vi "Get analysis parameters.vi"(6 "wait for reply (T)":bool=TRUE, 8 "error in":errorcluster) -> (0 "error out":errorcluster, 1 "timed out?":bool, 2 "Decimation":T2={"App"={"Dec"=1, "apply"=FALSE}, "Con"={"Dec"=1, "apply"=FALSE}, "Ret"={"Dec"=1, "apply"=FALSE}}, 3 "Contact":T3, 4 "Tau Delay (ms)":dbl, 5 "Savitzksky-Golay":T1)   [LabVIEW 2019, in "Main UI.lvlib"]
doc: "Gets the analysis parameters\n_____\nCreated using DQMH Event Scripter 6.1.0.128."
uses:
  Main UI.lvlib
  Main UI Shared/Decimation input --cluster.ctl
  Get analysis parameters Argument--cluster.ctl
  Get analysis parameters (Reply Payload)--cluster.ctl
  Main UI Shared/MAIN UI Shared.lvlib
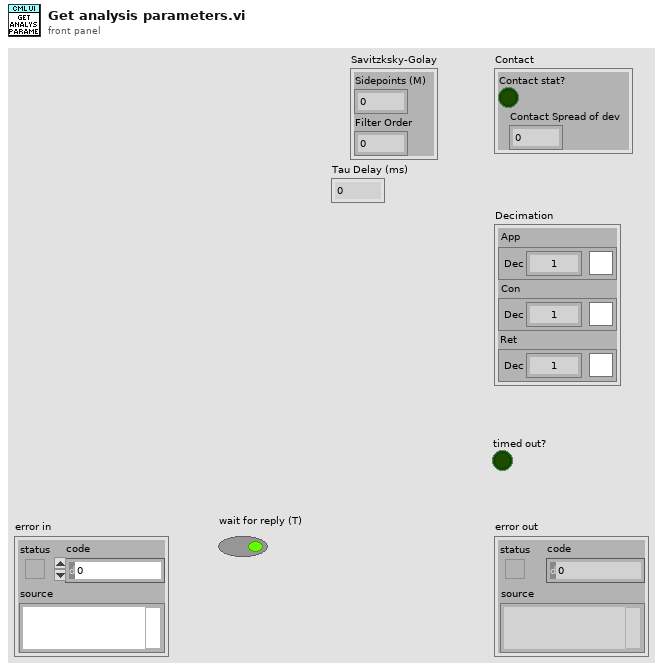
[diagram p1: front panel]
types:
  T1 = cluster{"Sidepoints (M)":dbl, "Filter Order":i32}
  T2 = typedef "MAIN UI Shared.lvlib/Decimation input --cluster.ctl" = cluster{"App":cluster{"Dec":i32, "apply":bool}, "Con":cluster{"Dec":i32, "apply":bool}, "Ret":cluster{"Dec":i32, "apply":bool}}
  T3 = cluster{"Contact stat?":bool, "Contact Spread of dev":dbl}
  T4 = typedef "Main UI.lvlib/Get analysis parameters Argument--cluster.ctl" = cluster{"Wait Notifier":refnum<notifier>, "wait for reply":bool}
  T5 = typedef "Main UI.lvlib/Request Events--cluster.ctl" = cluster{"Stop Module":refnum<user-event>, "Show Panel":refnum<user-event>, "Hide Panel":refnum<user-event>, "Get Module Execution Status":refnum<user-event>, "Show Diagram":refnum<user-event>, "Get analysis parameters":refnum<user-event>}
  T6 = typedef "Main UI.lvlib/Get analysis parameters (Reply Payload)--cluster.ctl" = cluster{"Contact":cluster{"Contact stat?":bool, "Contact Spread of dev":dbl}, "Decimation":T2, "Savitzksky-Golay":cluster{"Sidepoints (M)":dbl, "Filter Order":i32}, "Tau Delay (ms)":dbl, "error":errorcluster}
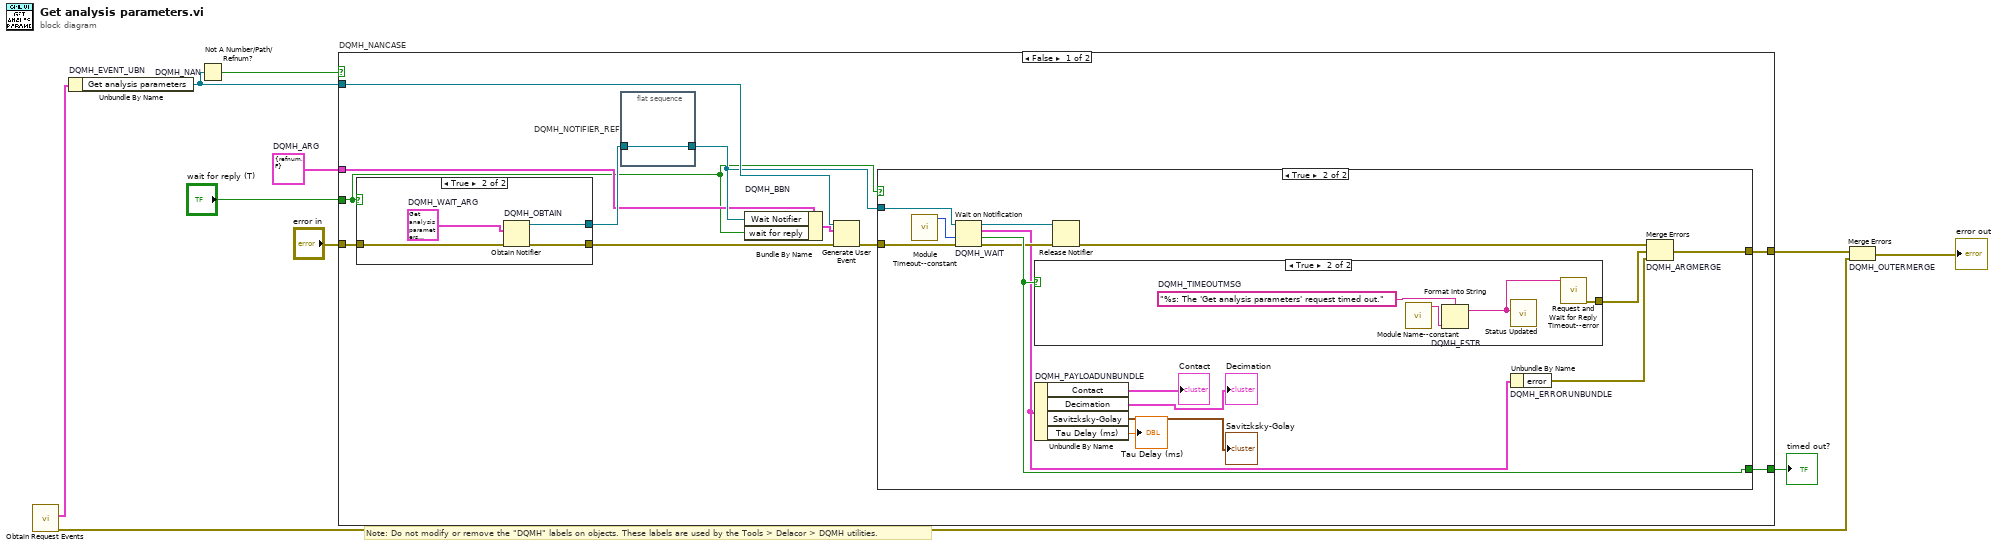
[diagram p0: block diagram]
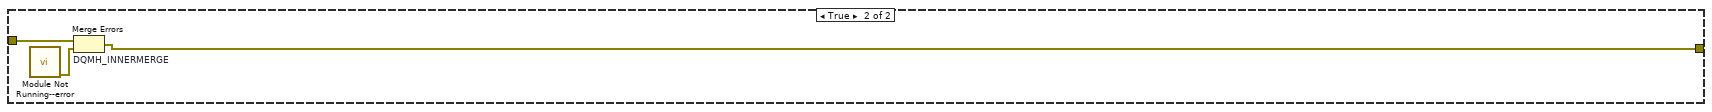
[diagram p5: hidden frame]
diagram:
  w4 = T4 {"Wait Notifier"=refnum, "wait for reply"=FALSE}  # DQMH_ARG
  # "Note: Do not modify or remove the \"DQMH\" labels on objects. These labels are used by the Tools > Delacor > DQMH utilities."
  n1 = call "Obtain Request Events.vi"() -> ("error out"=w2:errorcluster, "Main UI Request Events"=w1:T5)  [unwired: 10 in]
  n2 = Unbundle By Name "DQMH_EVENT_UBN"(w1) -> ("Get analysis parameters"=w8:refnum<user-event>)
  n3 = Not A Number/Path/Refnum? "DQMH_NAN"(number/path/refnum=w8) -> (NaN/Path/Refnum?=w7:bool)
  n4 = case "DQMH_NANCASE" shown="False" w7 {
    tunnel: "error in" -> [w21 w50]
    tunnel: w8 -> [w19 _]
    tunnel: [w16 w49] -> w5
    tunnel: [w17 _] -> w6
    tunnel: w4 -> [w12 _]
    tunnel: "wait for reply (T)" -> [w11 _]
    frame False {
      n5 = case shown="True" w11 {
        tunnel: w21 -> [w43 w47]
        tunnel: [w43 w46] -> w18
        tunnel: [_ w44] -> w14
        frame False {
        }
        frame True {
          w45 = T6 {"Contact"={"Contact stat?"=TRUE, "Contact Spread of dev"=0.0}, "Decimation"={"App"={"Dec"=1, "apply"=FALSE}, "Con"={"Dec"=1, "apply"=FALSE}, "Ret"={"Dec"=1, "apply"=FALSE}}, "Savitzksky-Golay"={"Sidepoints (M)"=20.0, "Filter Order"=5}, "Tau Delay (ms)"=0.0, "error"={"status"=FALSE, "code"=0, "source"=""}}  # DQMH_WAIT_ARG
          n6 = Obtain Notifier "DQMH_OBTAIN"(notification data type=w45, error in (no error)=w47) -> (notifier out=w44:refnum<notifier>, error out=w46:errorcluster)  [unwired: 2 in, 1 out]
        }
      }
      n7 = flat-sequence "DQMH_NOTIFIER_REF" {
        tunnel: w14 -> [w22]
        tunnel: [w22] -> w13
        frame #0 {
        }
      }
      n8 = Bundle By Name "DQMH_BBN"(cluster=w12, "Wait Notifier"=w13, "wait for reply"=w11) -> (w15:T4)
      n9 = Generate User Event(user event=w19, event data cluster=w15, error in=w18) -> (error out=w20:errorcluster)  [unwired: 1 in, 1 out]
      n10 = case shown="True" w11 {
        tunnel: w20 -> [w23 w38]
        tunnel: w13 -> [_ w37]
        tunnel: [_ w35] -> w17
        tunnel: [w23 w34] -> w16
        frame False {
        }
        frame True {
          n11 = call "Module Timeout--constant.vi"() -> ("Module Timeout"=w28:i32)  [unwired: 11 in]
          n12 = Wait on Notification "DQMH_WAIT"(notifier=w37, timeout in ms (-1)=w28, error in (no error)=w38) -> (notifier out=w36:refnum<notifier>, notification=w29:T6, timed out?=w35:bool, error out=w33:errorcluster)  [unwired: 1 in]
          n13 = case shown="True" w35 {
            tunnel: [_ w40] -> w30
            frame False {
            }
            frame True {
              w42 = "%s: The 'Get analysis parameters' request timed out."  # DQMH_TIMEOUTMSG
              n14 = call "Module Name--constant.vi"() -> ("Module Name"=w39:string)  [unwired: 11 in]
              n15 = Format Into String "DQMH_FSTR"(format string=w42, w39) -> (resulting string=w41:string)  [unwired: 2 in, 1 out]
              n16 = call "Status Updated.vi"("Status"=w41) -> ()  [unwired: 10 in, 1 out]
              n17 = call "Request and Wait for Reply Timeout--error.vi"("Error Message"=w41) -> ("error out"=w40:errorcluster)  [unwired: 10 in]
            }
          }
          n18 = Unbundle By Name "DQMH_PAYLOADUNBUNDLE"(w29) -> ("Contact"=→"Contact":T3, "Decimation"=→"Decimation":T2, "Savitzksky-Golay"=→"Savitzksky-Golay":T1, "Tau Delay (ms)"=→"Tau Delay (ms)":dbl)
          n19 = Release Notifier(notifier=w36, error in (no error)=w33) -> (error out=w32:errorcluster)  [unwired: 1 in, 2 out]
          n20 = Unbundle By Name "DQMH_ERRORUNBUNDLE"(w29) -> ("error"=w31:errorcluster)
          n21 = Merge Errors "DQMH_ARGMERGE"(w32, w30, w31) -> (w34:errorcluster)
        }
      }
    }
    frame True {
      n22 = call "Module Not Running--error.vi"() -> ("error out"=w48:errorcluster)  [unwired: 11 in]
      n23 = Merge Errors "DQMH_INNERMERGE"(w50, w48) -> (w49:errorcluster)
    }
  }
  "timed out?" <- w6
  n24 = Merge Errors "DQMH_OUTERMERGE"(w5, w2) -> (→"error out":errorcluster)
